vi "Autonomous Independent.vi"   [LabVIEW 2011]
doc: "This VI is called when autonomous begins, and will automatically be terminated when autonomous ends. You can carry out timed or sensor driven robot movement independently without needing to return to the caller."
uses:
  Robot Global Data.vi
types:
  T1 = typedef "WPI_MotorControlDeviceRef.ctl" = cluster{"DeviceStatus":errorcluster, "Type":enum16{"PWM", "CAN"}, "PWM":cluster{"Digital Module":T2, "PWM Channel":T3, "DeadBand":T4}, "CAN":cluster{"Device Number":u8, "Control Mode":T5, "Semaphore":T6, "Max Vout":dbl}, "Invert":bool, "TransformRef":T7, "InvTransformRef":T7}
  T2 = typedef "FPGA_TypedefDigitalModule.ctl" = enum16{"Digital Module 1", "Digital Module 2"}
  T3 = typedef "FPGA_DIOPWMChannel.ctl" = enum8{"PWM 1", "PWM 2", "PWM 3", "PWM 4", "PWM 5", "PWM 6", "PWM 7", "PWM 8", "PWM 9", "PWM 10", "Invalid"}
  T4 = typedef "WPI_PWMDeadband.ctl" = cluster{"Name":string, "maxPositivePwm":i32, "minPositivePwm":i32, "centerPwm":i32, "maxNegativePwm":i32, "minNegativePwm":i32, "angularRange":u16}
  T5 = typedef "WPI_CANJaguar_ControlMode.ctl" = enum8{"Percent VBus", "Current", "Speed", "Position", "Voltage"}
  T6 = typedef "Semaphore RefNum" = refnum<k1>
  T7 = typedef "WPI_PWMTransform_ConPane.ctl" = refnum<vi>
  T8 = typedef "WPI_DigitalInputDevRef.ctl" = cluster{"DevStatus":errorcluster, "DIO Channel":T9, "Digital Module":T2}
  T9 = typedef "FPGA_DIOChannel.ctl" = enum8{"DIO 1", "DIO 2", "DIO 3", "DIO 4", "DIO 5", "DIO 6", "DIO 7", "DIO 8", "DIO 9", "DIO 10", "DIO 11", "DIO 12", "DIO 13", "DIO 14", "Invalid"}
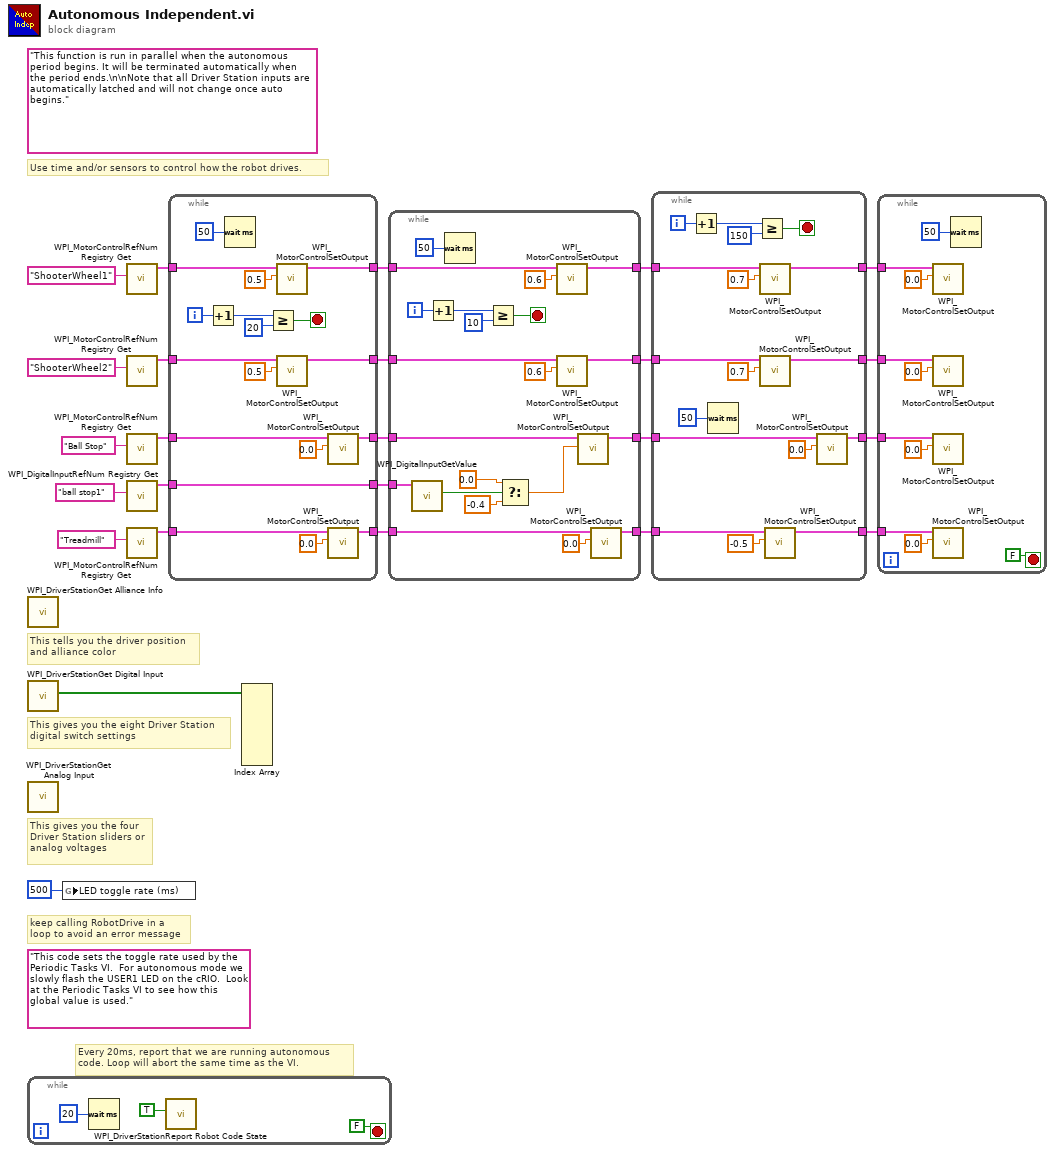
[diagram p0: block diagram]
diagram:
  (unwired) "This code sets the toggle rate used by the Periodic Tasks VI.  For autonomous mode we slowly flash the USER1 LED on the cRIO.  Look at the Periodic Tasks VI to see how this global value is used."
  (unwired) "This function is run in parallel when the autonomous period begins. It will be terminated automatically when the period ends.\n\nNote that all Driver Station inputs are automatically latched and will not change once auto begins."
  # "keep calling RobotDrive in a loop to avoid an error message"
  # "Every 20ms, report that we are running autonomous\ncode. Loop will abort the same time as the VI."
  # "Use time and/or sensors to control how the robot drives."
  # "This tells you the driver position\nand alliance color"
  # "This gives you the eight Driver Station\ndigital switch settings"
  # "This gives you the four\nDriver Station sliders or\nanalog voltages"
  n1 = call <vilib>:"WPI_DriverStationGet Alliance Info.vi"() -> ()  [unwired: 12 out]
  n2 = call <vilib>:"WPI_DriverStationGet Digital Input.vi"() -> ("Driver Station Digital Input (1-8)"=w25:bool[])  [unwired: 11 out]
  n3 = call <vilib>:"WPI_DriverStationGet Analog Input.vi"() -> ()  [unwired: 12 out]
  n4 = while {
    stop <- FALSE stop-if-true
    n5 = Wait (ms)(milliseconds to wait=u32 20) -> ()  [unwired: 1 out]
    n6 = call <vilib>:"WPI_DriverStationReport Robot Code State.vi"("Autonomous"=TRUE) -> ()  [unwired: 10 in, 1 out]
  }
  n7 = global write "Robot Global Data.vi" "LED toggle rate (ms)"(u32 500 ("LED ms toggle rate")) -> ()
  n8 = call <vilib>:"WPI_MotorControlRefNum Registry Get.vi"("refnum name"="ShooterWheel1") -> ("MotorControlDevRef"=w22:T1)  [unwired: 9 in, 1 out]
  n9 = call <vilib>:"WPI_MotorControlRefNum Registry Get.vi"("refnum name"="ShooterWheel2") -> ("MotorControlDevRef"=w23:T1)  [unwired: 9 in, 1 out]
  n10 = call <vilib>:"WPI_MotorControlRefNum Registry Get.vi"("refnum name"="Ball Stop") -> ("MotorControlDevRef"=w17:T1)  [unwired: 9 in, 1 out]
  n11 = call <vilib>:"WPI_DigitalInputRefNum Registry Get.vi"("refnum name"="ball stop1") -> ("DigitalInputDevRef"=w1:T8)  [unwired: 9 in, 1 out]
  n12 = call <vilib>:"WPI_MotorControlRefNum Registry Get.vi"("refnum name"="Treadmill") -> ("MotorControlDevRef"=w16:T1)  [unwired: 9 in, 1 out]
  n13 = while {
    tunnel: w23 -> [w40]
    tunnel: w22 -> [w38]
    tunnel: [w37] -> w19
    tunnel: [w36] -> w18
    tunnel: w17 -> [w35]
    tunnel: w16 -> [w34]
    tunnel: [w31] -> w15
    tunnel: [w30] -> w14
    tunnel: [w29] -> w2
    tunnel: w1 -> [w29]
    i -> [w45]
    stop <- w43 stop-if-true
    n14 = Increment(x=w45) -> (x+1=w42:i32)
    n15 = Wait (ms)(milliseconds to wait=u32 50) -> ()  [unwired: 1 out]
    n16 = Greater Or Equal?(x=w42, y=20) -> (x >= y?=w43:bool)
    n17 = call <vilib>:"WPI_MotorControlSetOutput.vi"("Output"=0.5, "MotorControlDevRef"=w38) -> ("MotorControlDevRef"=w36:T1)  [unwired: 8 in, 1 out]
    n18 = call <vilib>:"WPI_MotorControlSetOutput.vi"("Output"=0.5, "MotorControlDevRef"=w40) -> ("MotorControlDevRef"=w37:T1)  [unwired: 8 in, 1 out]
    n19 = call <vilib>:"WPI_MotorControlSetOutput.vi"("Output"=0.0, "MotorControlDevRef"=w35) -> ("MotorControlDevRef"=w31:T1)  [unwired: 8 in, 1 out]
    n20 = call <vilib>:"WPI_MotorControlSetOutput.vi"("Output"=0.0, "MotorControlDevRef"=w34) -> ("MotorControlDevRef"=w30:T1)  [unwired: 8 in, 1 out]
  }
  n21 = Index Array(array=w25) -> ()  [unwired: 8 in, 8 out]
  n22 = while {
    tunnel: w19 -> [w60]
    tunnel: w18 -> [w55]
    tunnel: w15 -> [w59]
    tunnel: w14 -> [w58]
    tunnel: [w56] -> w13
    tunnel: [w54] -> w12
    tunnel: [w53] -> w11
    tunnel: [w52] -> w10
    tunnel: w2 -> [w51]
    i -> [w66]
    stop <- w64 stop-if-true
    n23 = call <vilib>:"WPI_DigitalInputGetValue.vi"("DigitalInputDevRef"=w51) -> ("Value"=w50:bool)  [unwired: 8 in, 2 out]
    n24 = Increment(x=w66) -> (x+1=w63:i32)
    n25 = Wait (ms)(milliseconds to wait=u32 50) -> ()  [unwired: 1 out]
    n26 = Greater Or Equal?(x=w63, y=10) -> (x >= y?=w64:bool)
    n27 = Select(t=0.0, s=w50, f=-0.4 ("Output")) -> (s? t:f=w49:dbl)
    n28 = call <vilib>:"WPI_MotorControlSetOutput.vi"("Output"=0.6, "MotorControlDevRef"=w55) -> ("MotorControlDevRef"=w53:T1)  [unwired: 8 in, 1 out]
    n29 = call <vilib>:"WPI_MotorControlSetOutput.vi"("Output"=0.6, "MotorControlDevRef"=w60) -> ("MotorControlDevRef"=w54:T1)  [unwired: 8 in, 1 out]
    n30 = call <vilib>:"WPI_MotorControlSetOutput.vi"("Output"=w49, "MotorControlDevRef"=w59) -> ("MotorControlDevRef"=w56:T1)  [unwired: 8 in, 1 out]
    n31 = call <vilib>:"WPI_MotorControlSetOutput.vi"("Output"=0.0, "MotorControlDevRef"=w58) -> ("MotorControlDevRef"=w52:T1)  [unwired: 8 in, 1 out]
  }
  n32 = while {
    tunnel: w13 -> [w83]
    tunnel: w12 -> [w80]
    tunnel: w11 -> [w77]
    tunnel: w10 -> [w76]
    tunnel: [w71] -> w9
    tunnel: [w70] -> w8
    tunnel: [w69] -> w7
    tunnel: [w68] -> w6
    i -> [w73]
    stop <- w72 stop-if-true
    n33 = Increment(x=w73) -> (x+1=w74:i32)
    n34 = Wait (ms)(milliseconds to wait=u32 50) -> ()  [unwired: 1 out]
    n35 = Greater Or Equal?(x=w74, y=150) -> (x >= y?=w72:bool)
    n36 = call <vilib>:"WPI_MotorControlSetOutput.vi"("Output"=0.7, "MotorControlDevRef"=w77) -> ("MotorControlDevRef"=w71:T1)  [unwired: 8 in, 1 out]
    n37 = call <vilib>:"WPI_MotorControlSetOutput.vi"("Output"=0.7, "MotorControlDevRef"=w80) -> ("MotorControlDevRef"=w70:T1)  [unwired: 8 in, 1 out]
    n38 = call <vilib>:"WPI_MotorControlSetOutput.vi"("Output"=-0.5, "MotorControlDevRef"=w76) -> ("MotorControlDevRef"=w69:T1)  [unwired: 8 in, 1 out]
    n39 = call <vilib>:"WPI_MotorControlSetOutput.vi"("Output"=0.0, "MotorControlDevRef"=w83) -> ("MotorControlDevRef"=w68:T1)  [unwired: 8 in, 1 out]
  }
  n40 = while {
    tunnel: w9 -> [w93]
    tunnel: w8 -> [w92]
    tunnel: w7 -> [w91]
    tunnel: w6 -> [w90]
    stop <- FALSE stop-if-true
    n41 = call <vilib>:"WPI_MotorControlSetOutput.vi"("Output"=0.0, "MotorControlDevRef"=w93) -> ()  [unwired: 8 in, 2 out]
    n42 = call <vilib>:"WPI_MotorControlSetOutput.vi"("Output"=0.0, "MotorControlDevRef"=w92) -> ()  [unwired: 8 in, 2 out]
    n43 = call <vilib>:"WPI_MotorControlSetOutput.vi"("Output"=0.0, "MotorControlDevRef"=w90) -> ()  [unwired: 8 in, 2 out]
    n44 = call <vilib>:"WPI_MotorControlSetOutput.vi"("Output"=0.0, "MotorControlDevRef"=w91) -> ()  [unwired: 8 in, 2 out]
    n45 = Wait (ms)(milliseconds to wait=u32 50) -> ()  [unwired: 1 out]
  }
